vi "set UI state when stop line.vi"(9 "index of element":i32, 10 "UI Refs":T1) -> ()   [LabVIEW 2014]
uses:
  controls/PLS UI Data.ctl
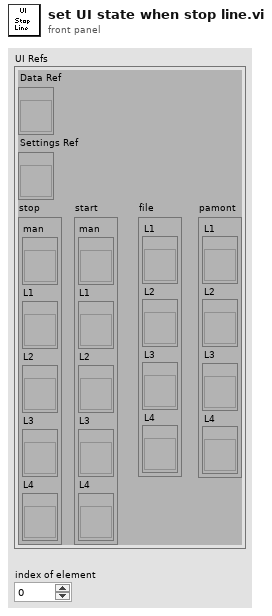
[diagram p1: front panel]
types:
  T1 = typedef "PLS UI Data.ctl" = cluster{"Data Ref":refnum<vi>, "Settings Ref":refnum<vi>, "stop":cluster{"man":refnum<vi>, "L1":refnum<vi>, "L2":refnum<vi>, "L3":refnum<vi>, "L4":refnum<vi>}, "start":cluster{"man":refnum<vi>, "L1":refnum<vi>, "L2":refnum<vi>, "L3":refnum<vi>, "L4":refnum<vi>}, "file":cluster{"L1":refnum<vi>, "L2":refnum<vi>, "L3":refnum<vi>, "L4":refnum<vi>}, "pamont":cluster{"L1":refnum<vi>, "L2":refnum<vi>, "L3":refnum<vi>, "L4":refnum<vi>}}
  T2 = cluster{"L1":refnum<vi>, "L2":refnum<vi>, "L3":refnum<vi>, "L4":refnum<vi>}
  T3 = cluster{"man":refnum<vi>, "L1":refnum<vi>, "L2":refnum<vi>, "L3":refnum<vi>, "L4":refnum<vi>}
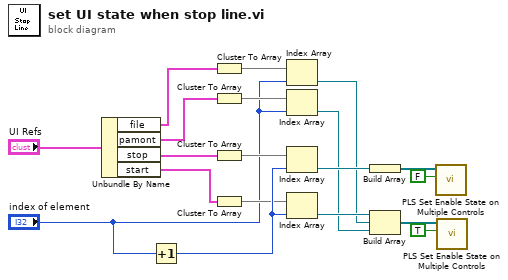
[diagram p0: block diagram]
diagram:
  n1 = Unbundle By Name("UI Refs") -> ("file"=w5:T2, "pamont"=w4:T2, "stop"=w11:T3, "start"=w12:T3)
  n2 = Increment(x="index of element") -> (x+1=w15:i32)
  n3 = Cluster To Array(cluster=w5) -> (array=w6:refnum<vi>[])
  n4 = Cluster To Array(cluster=w4) -> (array=w7:refnum<vi>[])
  n5 = Cluster To Array(cluster=w11) -> (array=w14:refnum<vi>[])
  n6 = Cluster To Array(cluster=w12) -> (array=w13:refnum<vi>[])
  n7 = Index Array(array=w6, index="index of element") -> (element=w2:refnum<vi>)
  n8 = Index Array(array=w7, index="index of element") -> (element=w1:refnum<vi>)
  n9 = Index Array(array=w14, index=w15) -> (element=w16:refnum<vi>)
  n10 = Index Array(array=w13, index=w15) -> (element=w18:refnum<vi>)
  n11 = Build Array(w16) -> (w17:refnum<vi>[])
  n12 = Build Array(w18, w2, w1) -> (w19:refnum<vi>[])
  n13 = call "PLS Set Enable State on Multiple Controls.vi"("Enable?"=FALSE, "Controls"=w17) -> ()  [unwired: 10 in]
  n14 = call "PLS Set Enable State on Multiple Controls.vi"("Enable?"=TRUE, "Controls"=w19) -> ()  [unwired: 10 in]
